vi "UpdateOdorConcInf.vi"(9 "Path":path, 10 "Concentration Ref":refnum<vi>, 11 "Odor Ref":refnum<vi>) -> ()   [LabVIEW 2016]
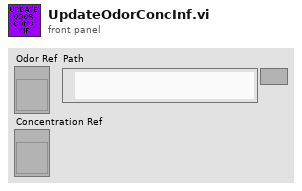
[diagram p1: front panel]
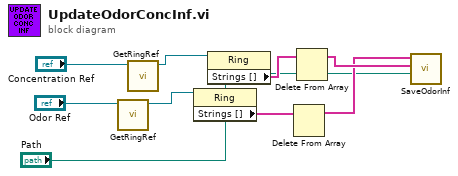
[diagram p0: block diagram]
diagram:
  n1 = call "GetRingRef.vi"("Array Reference"="Odor Ref") -> ("Ring Reference"=w8:refnum<vi>)  [unwired: 9 in, 1 out]
  n2 = call "GetRingRef.vi"("Array Reference"="Concentration Ref") -> ("Ring Reference"=w9:refnum<vi>)  [unwired: 9 in, 1 out]
  n3 = property class="Ring"(reference=w8) -> ("Strings []"=w6:string[])  [unwired: 1 in, 2 out]
  n4 = property class="Ring"(reference=w9) -> ("Strings []"=w7:string[])  [unwired: 1 in, 2 out]
  n5 = Delete From Array(array=w6) -> (array with subset deleted=w4:string[])  [unwired: 2 in, 1 out]
  n6 = Delete From Array(array=w7) -> (array with subset deleted=w5:string[])  [unwired: 2 in, 1 out]
  n7 = call "SaveOdorInf.vi"("Path"="Path", "Concentrations"=w5, "Odors"=w4) -> ()  [unwired: 9 in]
